vi "dsmm-test.vi"() -> ()   [LabVIEW 2017]
uses:
  <vilib>/Utility/file.llb/Read Delimited Spreadsheet (DBL).vi
panel:
  in  "lambda":dbl=1.5
  in  "beta":dbl=3.0
  in  "eq_tol":dbl=0.001 format="%#_13g"
  in  "conv_epsilon":dbl=0.001 format="%#_13g"
  out "avg exec time":dbl
  out "XY Graph":cluster{dbl[], dbl[]}[](graph)
  in  "Y":string="C:\\Users\\francesco\\dev\\pointsetregistrations\\data\\fish_Y.txt"
  in  "X":string="C:\\Users\\francesco\\dev\\pointsetregistrations\\data\\fish_X.txt"
  # "s"
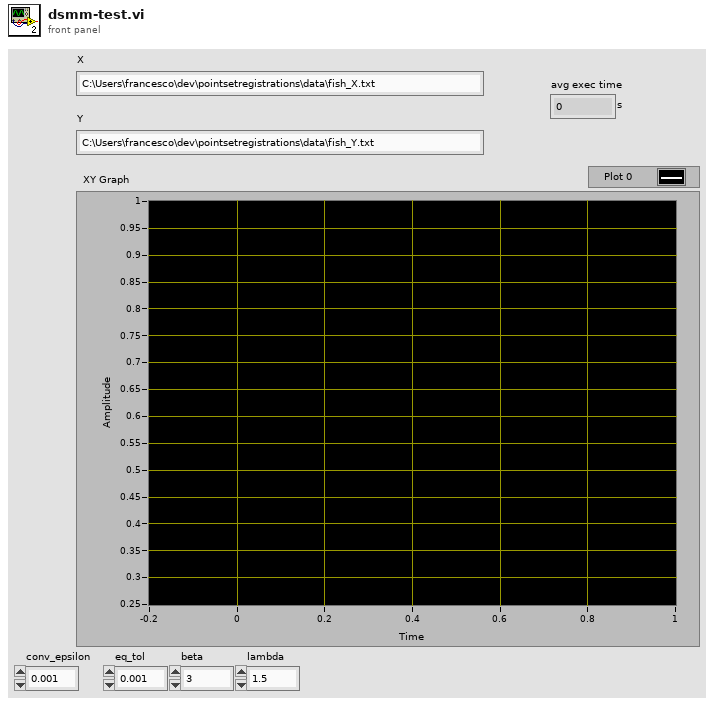
[diagram p1: front panel]
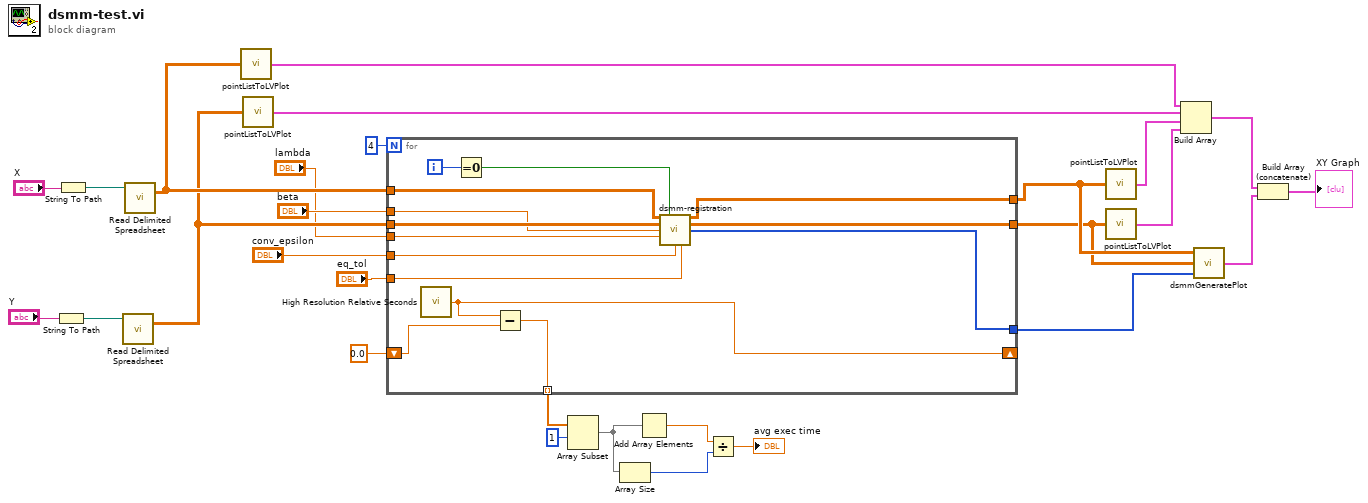
[diagram p0: block diagram]
diagram:
  n1 = String To Path(string="Y") -> (path=w26:path)
  n2 = String To Path(string="X") -> (path=w27:path)
  n3 = call-poly <vilib>:"Read Delimited Spreadsheet.vi"("file path (dialog if empty)"=w26) -> ("all rows"=w22:dbl[][])  [unwired: 9 in, 5 out]
  n4 = call-poly <vilib>:"Read Delimited Spreadsheet.vi"("file path (dialog if empty)"=w27) -> ("all rows"=w23:dbl[][])  [unwired: 9 in, 5 out]
  n5 = call "pointListToLVPlot.vi"("XY[N,d]"=w23) -> ("LV plot"=w24:cluster{dbl[], dbl[]})
  n6 = call "pointListToLVPlot.vi"("XY[N,d]"=w22) -> ("LV plot"=w21:cluster{dbl[], dbl[]})
  n7 = for {
    N: 4 -> [_]
    tunnel: w23 -> [w42]
    tunnel: w22 -> [w41]
    tunnel: [w40] -> w3
    shift-right: [w38] -> _
    shift-left: 0.0 -> [w39]
    tunnel: [w37] -> w18 mode=indexing
    tunnel: [w34] -> w4
    tunnel: "conv_epsilon" -> [w33]
    tunnel: "eq_tol" -> [w32]
    tunnel: [w31] -> w2
    tunnel: "beta" -> [w30]
    tunnel: "lambda" -> [w29]
    i -> [w36]
    n8 = call <vilib>:"High Resolution Relative Seconds.vi"() -> ("relative seconds"=w38:dbl)
    n9 = Equal To 0?(x=w36) -> (x = 0?=w35:bool)
    n10 = Subtract(x=w38, y=w39) -> (x-y=w37:dbl)
    n11 = call "dsmm-registration.vi"("X"=w42, "allocate"=w35, "Y"=w41, "beta"=w30, "lambda"=w29, "conv_epsilon"=w33, "eq_tol"=w32) -> ("X out"=w34:dbl[][], "Y out"=w40:dbl[][], "Match"=w31:i32[])  [unwired: 5 in, 1 out]
  }
  n12 = Array Subset(array=w18, index=1) -> (w16:dbl[])  [unwired: 1 in]
  n13 = Array Size(array=w16) -> (size(s)=w14:i32)
  n14 = Add Array Elements(numeric array=w16) -> (sum=w15:dbl)
  n15 = Divide(x=w15, y=w14) -> (x/y=→"avg exec time":dbl)
  n16 = call "pointListToLVPlot.vi"("XY[N,d]"=w4) -> ("LV plot"=w12:cluster{dbl[], dbl[]})
  n17 = call "pointListToLVPlot.vi"("XY[N,d]"=w3) -> ("LV plot"=w11:cluster{dbl[], dbl[]})
  n18 = Build Array(w24, w21, w12, w11) -> (w8:cluster{dbl[], dbl[]}[])
  n19 = call "dsmmGeneratePlot.vi"("Match"=w2, "Y"=w3, "X"=w4) -> ("LV plot"=w1:cluster{dbl[], dbl[]}[])
  n20 = Build Array (concatenate)(w8, w1) -> (→"XY Graph":cluster{dbl[], dbl[]}[])
